vi "Search.vi"(8 "error in (no error)":errorcluster, 9 "SearchMethod":T1, 11 "Graph in":refnum<class "Graph.lvclass">) -> (0 "error out":errorcluster, 1 "found":bool, 2 "Node":refnum<data-value>, 3 "Graph out":refnum<class "Graph.lvclass">)   [LabVIEW 2013, in "Graph.lvclass"]
doc: "Searches the graph based on method choosen."
uses:
  Graph.lvclass
  SearchMethod.ctl
  GraphNode/GraphNode.lvclass
  Graph.lvclass/Graph.ctl
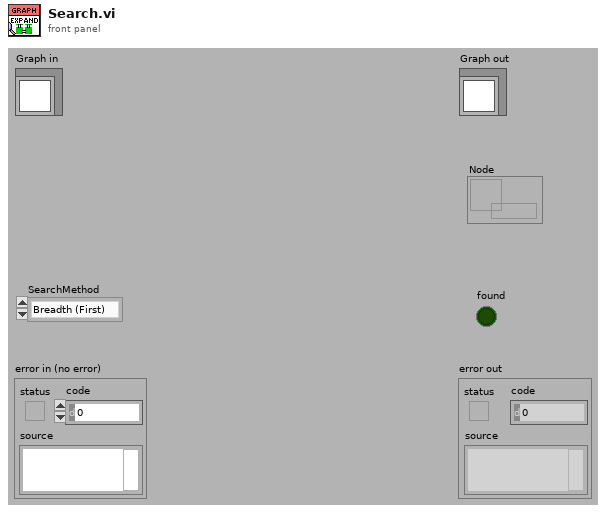
[diagram p1: front panel]
types:
  T1 = typedef "Graph.lvclass/SearchMethod.ctl" = enum16{"Breadth (First)", "Depth (First)", "Best First", "Breadth (Best)", "Depth (Best)"}
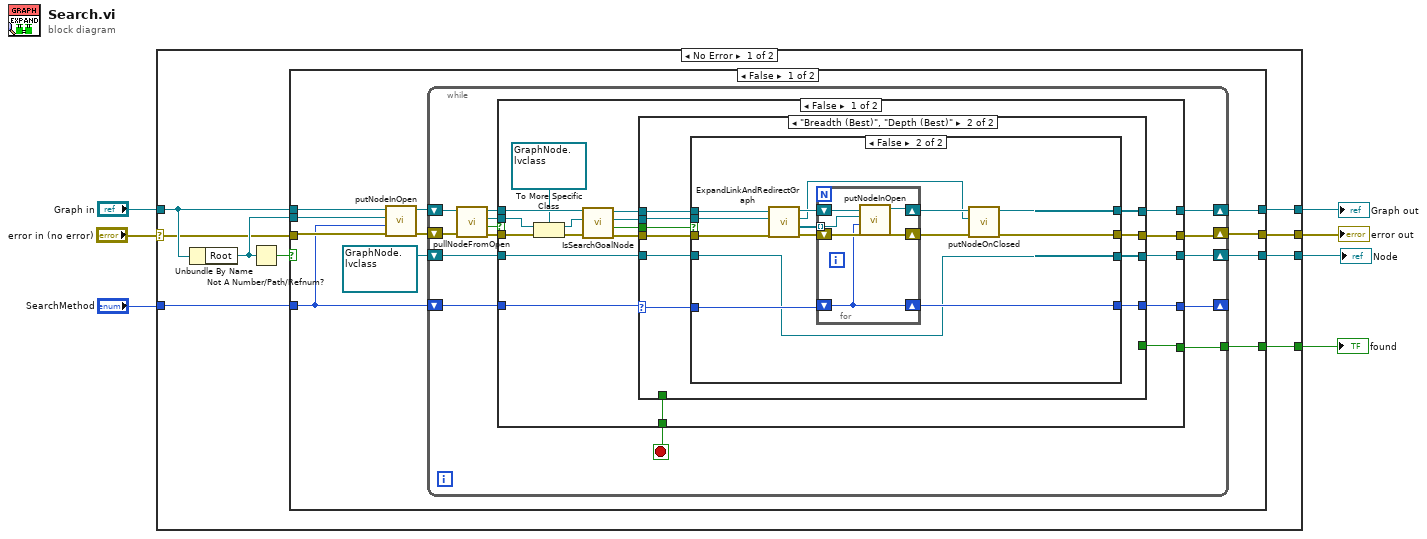
[diagram p0: block diagram]
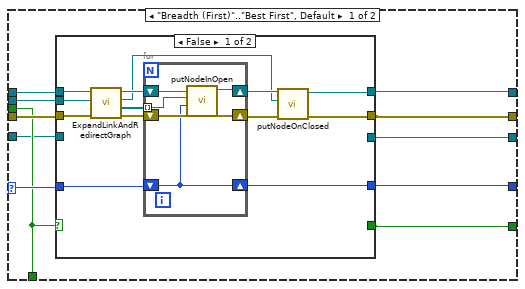
[diagram p2: hidden frame]
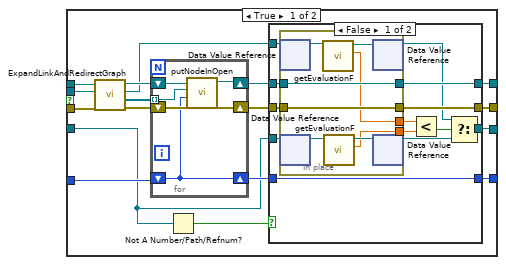
[diagram p4: hidden frame]
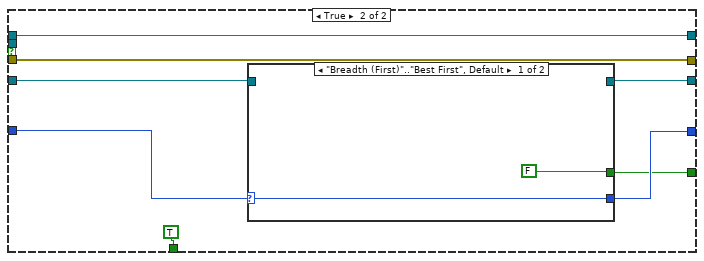
[diagram p6: hidden frame]
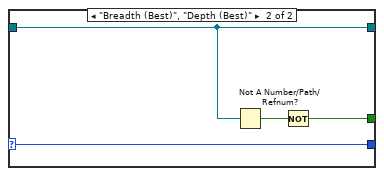
[diagram p7: hidden frame]
diagram:
  n1 = case shown="No Error" "error in (no error)" {
    selector: "error in (no error)" -> [w13 w190]
    tunnel: [w11 w190] -> w2
    tunnel: [w12 w189] -> w1
    tunnel: "Graph in" -> [w15 w189]
    tunnel: [w10 _] -> w4
    tunnel: "SearchMethod" -> [w9 _]
    tunnel: [w8 _] -> w3
    frame No Error {
      n2 = Unbundle By Name(w15) -> ("Root"=w14:refnum<data-value>)
      n3 = Not A Number/Path/Refnum?(number/path/refnum=w14) -> (NaN/Path/Refnum?=w16:bool)
      n4 = case shown="False" w16 {
        tunnel: w15 -> [w27 w187]
        tunnel: w14 -> [w25 _]
        tunnel: w13 -> [w24 w188]
        tunnel: [w21 w187] -> w12
        tunnel: [w20 w188] -> w11
        tunnel: [w22 _] -> w10
        tunnel: w9 -> [w18 _]
        tunnel: [w19 _] -> w8
        frame False {
          n5 = call "putNodeInOpen.vi"("error in (no error)"=w24, "SearchMethod"=w18, "GraphNode"=w25, "Graph in"=w27) -> ("error out"=w23:errorcluster, "Graph out"=w26:refnum<class "Graph.lvclass">)  [unwired: 6 in]
          n6 = while {
            shift-right: [w34] -> w21
            shift-left: w26 -> [w40]
            shift-right: [w33] -> w20
            shift-left: w23 -> [w41]
            tunnel: [w35] -> w22
            shift-right: [w30] -> _
            shift-left: w18 -> [w31]
            shift-right: [w32] -> w19
            shift-left: refnum<data-value> refnum ("GraphNode out") -> [w28]
            stop <- w38 stop-if-true
            n7 = call "pullNodeFromOpen.vi"("error in (no error)"=w41, "Graph in"=w40) -> ("error out"=w39:errorcluster, "empty"=w37:bool, "RemovedNode"=w29:refnum<data-value>, "Graph out"=w36:refnum<class "Graph.lvclass">)  [unwired: 6 in]
            n8 = case shown="False" w37 {
              tunnel: w39 -> [w57 w178]
              tunnel: [w51 TRUE ("found")] -> w38
              tunnel: w36 -> [w59 w179]
              tunnel: [w43 w175] -> w35
              tunnel: [w45 w179] -> w34
              tunnel: [w46 w178] -> w33
              tunnel: [w44 w173] -> w32
              tunnel: w31 -> [w54 w177]
              tunnel: [w47 w176] -> w30
              tunnel: w29 -> [w58 _]
              tunnel: w28 -> [w53 w174]
              frame False {
                n9 = To More Specific Class(target class=refnum<data-value> refnum ("data value reference"), reference=w58, error in=w57) -> (specific class reference=w55:refnum<data-value>, error out=w56:errorcluster)
                n10 = call-dynamic "IsSearchGoalNode.vi"("error in (no error)"=w56, "PossibleGoalNode in"=w55, "Graph in"=w59) -> ("error out"=w50:errorcluster, "IsGoal"=w52:bool, "PossibleGoalNode out"=w49:refnum<data-value>, "Graph out"=w48:refnum<class "Graph.lvclass">)  [unwired: 5 in]
                n11 = case shown="\"Breadth (Best)\", \"Depth (Best)\"" w54 {
                  selector: w54 -> [w70 w103]
                  tunnel: [w65 w101] -> w47
                  tunnel: w53 -> [w61 w96]
                  tunnel: w52 -> [w62 w99]
                  tunnel: [w62 _] -> w51
                  tunnel: [w63 w95] -> w44
                  tunnel: w50 -> [w66 w100]
                  tunnel: w49 -> [w67 w102]
                  tunnel: w48 -> [w69 w104]
                  tunnel: [w68 w98] -> w45
                  tunnel: [w64 w97] -> w46
                  tunnel: [w60 _] -> w43
                  frame "Breadth (First)".."Best First", Default {
                    n12 = case shown="False" w62 {
                      selector: w62 -> [_ w94]
                      tunnel: [_ w94] -> w60
                      tunnel: w69 -> [w82 w93]
                      tunnel: [w74 w93] -> w68
                      tunnel: [w73 w91] -> w64
                      tunnel: w67 -> [w78 w90]
                      tunnel: w70 -> [w83 w92]
                      tunnel: [w77 w92] -> w65
                      tunnel: w66 -> [w76 w91]
                      tunnel: [_ w90] -> w63
                      tunnel: w61 -> [_ _]
                      frame False {
                        n13 = call "ExpandLinkAndRedirectGraph.vi"("error in (no error)"=w76, "GraphNode in"=w78, "Graph in"=w82) -> ("error out"=w80:errorcluster, "ExpandedNodes"=w79:refnum<data-value>[], "GraphNode out"=w71:refnum<data-value>, "Graph out"=w81:refnum<class "Graph.lvclass">)  [unwired: 5 in]
                        n14 = for {
                          shift-right: [w87] -> w75
                          shift-left: w81 -> [w89]
                          tunnel: w79 -> [w88] mode=indexing
                          shift-right: [w85] -> w72
                          shift-left: w80 -> [w86]
                          shift-right: [w84] -> w77
                          shift-left: w83 -> [w84]
                          n15 = call "putNodeInOpen.vi"("error in (no error)"=w86, "SearchMethod"=w84, "GraphNode"=w88, "Graph in"=w89) -> ("error out"=w85:errorcluster, "Graph out"=w87:refnum<class "Graph.lvclass">)  [unwired: 6 in]
                        }
                        n16 = call "putNodeOnClosed.vi"("error in (no error)"=w72, "GraphNode in"=w71, "Graph in"=w75) -> ("error out"=w73:errorcluster, "Graph out"=w74:refnum<class "Graph.lvclass">)  [unwired: 6 in, 1 out]
                      }
                      frame True {
                      }
                    }
                  }
                  frame "Breadth (Best)", "Depth (Best)" {
                    n17 = case shown="False" w99 {
                      tunnel: w104 -> [w118 w163]
                      tunnel: w103 -> [w117 w162]
                      tunnel: w102 -> [w116 w161]
                      tunnel: [w106 w160] -> w101
                      tunnel: w100 -> [w115 w159]
                      tunnel: [w111 w156] -> w98
                      tunnel: [w110 w155] -> w97
                      tunnel: w96 -> [w105 w158]
                      tunnel: [w109 w158] -> w95
                      frame True {
                        n18 = call "ExpandLinkAndRedirectGraph.vi"("error in (no error)"=w115, "GraphNode in"=w116, "Graph in"=w118) -> ("error out"=w120:errorcluster, "ExpandedNodes"=w119:refnum<data-value>[], "GraphNode out"=w114:refnum<data-value>, "Graph out"=w121:refnum<class "Graph.lvclass">)  [unwired: 5 in]
                        n19 = for {
                          shift-right: [w150] -> w112
                          shift-left: w121 -> [w152]
                          tunnel: w119 -> [w151] mode=indexing
                          shift-right: [w148] -> w113
                          shift-left: w120 -> [w149]
                          shift-right: [w147] -> w107
                          shift-left: w117 -> [w147]
                          n20 = call "putNodeInOpen.vi"("error in (no error)"=w149, "SearchMethod"=w147, "GraphNode"=w151, "Graph in"=w152) -> ("error out"=w148:errorcluster, "Graph out"=w150:refnum<class "Graph.lvclass">)  [unwired: 6 in]
                        }
                        n21 = Not A Number/Path/Refnum?(number/path/refnum=w105) -> (NaN/Path/Refnum?=w108:bool)
                        n22 = case shown="False" w108 {
                          tunnel: w114 -> [w134 w143]
                          tunnel: w113 -> [w133 w145]
                          tunnel: w112 -> [w132 w146]
                          tunnel: [w131 w146] -> w111
                          tunnel: [w130 w145] -> w110
                          tunnel: [w124 w143] -> w109
                          tunnel: w107 -> [w123 w144]
                          tunnel: [w123 w144] -> w106
                          tunnel: w105 -> [w122 _]
                          frame False {
                            n23 = in-place {
                              in-place-border: w133 -> [w138]
                              in-place-border: [w138] -> w130
                              in-place-border: w132 -> [w137]
                              in-place-border: [w137] -> w131
                              in-place-border: [w136] -> w129
                              in-place-border: [w135] -> w128
                              n24 = in-place-dvr #1(w134) -> (w142:refnum<class "GraphNode.lvclass">)  [unwired: 1 out]
                              n25 = in-place-dvr #2(w122) -> (w140:refnum<class "GraphNode.lvclass">)  [unwired: 1 out]
                              n26 = call "getEvaluationF.vi"("GraphNode in"=w142) -> ("F"=w136:dbl, "GraphNode out"=w141:refnum<class "GraphNode.lvclass">)  [unwired: 8 in, 1 out]
                              n27 = call "getEvaluationF.vi"("GraphNode in"=w140) -> ("F"=w135:dbl, "GraphNode out"=w139:refnum<class "GraphNode.lvclass">)  [unwired: 8 in, 1 out]
                              n28 = in-place-dvr #1(w141) -> (w126:refnum<data-value>)  [unwired: 1 out]
                              n29 = in-place-dvr #2(w139) -> (w125:refnum<data-value>)  [unwired: 1 out]
                            }
                            n30 = Less?(x=w129, y=w128) -> (x < y?=w127:bool)
                            n31 = Select(t=w126, s=w127, f=w125) -> (s? t:f=w124:refnum<data-value>)
                          }
                          frame True {
                          }
                        }
                      }
                      frame False {
                        n32 = call "ExpandLinkAndRedirectGraph.vi"("error in (no error)"=w159, "GraphNode in"=w161, "Graph in"=w163) -> ("error out"=w165:errorcluster, "ExpandedNodes"=w164:refnum<data-value>[], "GraphNode out"=w153:refnum<data-value>, "Graph out"=w166:refnum<class "Graph.lvclass">)  [unwired: 5 in]
                        n33 = for {
                          shift-right: [w170] -> w157
                          shift-left: w166 -> [w172]
                          tunnel: w164 -> [w171] mode=indexing
                          shift-right: [w168] -> w154
                          shift-left: w165 -> [w169]
                          shift-right: [w167] -> w160
                          shift-left: w162 -> [w167]
                          n34 = call "putNodeInOpen.vi"("error in (no error)"=w169, "SearchMethod"=w167, "GraphNode"=w171, "Graph in"=w172) -> ("error out"=w168:errorcluster, "Graph out"=w170:refnum<class "Graph.lvclass">)  [unwired: 6 in]
                        }
                        n35 = call "putNodeOnClosed.vi"("error in (no error)"=w154, "GraphNode in"=w153, "Graph in"=w157) -> ("error out"=w155:errorcluster, "Graph out"=w156:refnum<class "Graph.lvclass">)  [unwired: 6 in, 1 out]
                      }
                    }
                  }
                }
              }
              frame True {
                n36 = case shown="\"Breadth (First)\"..\"Best First\", Default" w177 {
                  selector: w177 -> [w182 w186]
                  tunnel: [w182 w186] -> w176
                  tunnel: [FALSE w183] -> w175
                  tunnel: w174 -> [_ w185]
                  tunnel: [_ w185] -> w173
                  frame "Breadth (First)".."Best First", Default {
                  }
                  frame "Breadth (Best)", "Depth (Best)" {
                    n37 = Not A Number/Path/Refnum?(number/path/refnum=w185) -> (NaN/Path/Refnum?=w184:bool)
                    n38 = Not(x=w184) -> (.not. x?=w183:bool)
                  }
                }
              }
            }
          }
        }
        frame True {
        }
      }
    }
    frame Error {
    }
  }
  "error out" <- w2
  "Graph out" <- w1
  "Node" <- w3
  "found" <- w4
